vi "Write Ramp Current.vi"(8 "error in":errorcluster, 10 "Current_Ramp":dbl, 11 "69X_79X in":refnum<class "7976A.lvclass">) -> (0 "error out":errorcluster, 3 "69X_79X out":refnum<class "7976A.lvclass">)   [LabVIEW 2019, in "7976A.lvlib" / "7976A.lvclass"]
uses:
  Library/7976A.lvclass
  C:/Users/Public/Documents/Development/builds/Instruments/PowerSupply.lvlibp/Library/PowerSupply.lvclass
  builds/Instruments/PowerSupply.lvlibp/Library/PowerSupply.lvclass
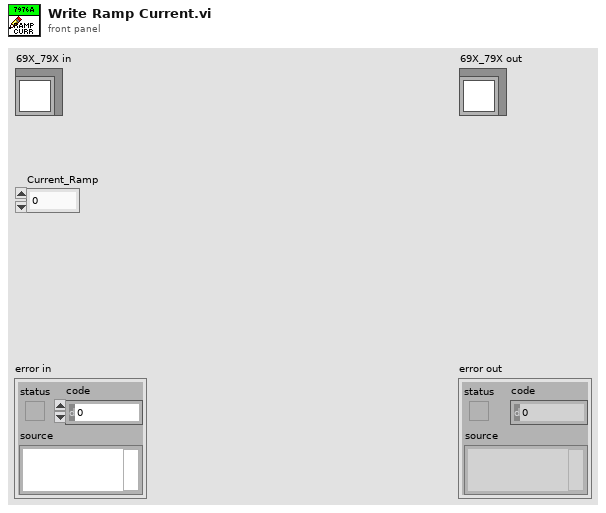
[diagram p1: front panel]
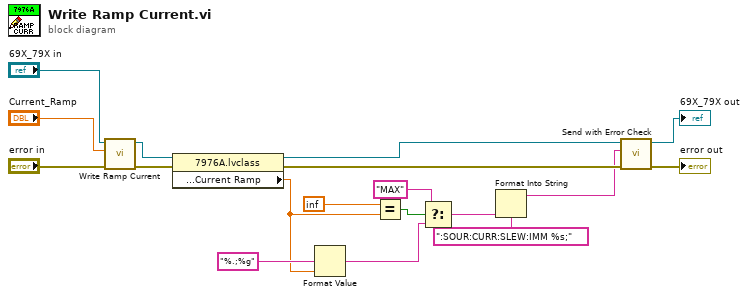
[diagram p0: block diagram]
diagram:
  n1 = call-parent "Write Ramp Current.vi"("error in"="error in", "Current_Ramp"="Current_Ramp", "PowerSupply in"="69X_79X in") -> ("error out"=w15:errorcluster, "PowerSupply out"=w11:refnum<class "7976A.lvclass">)  [unwired: 7 in]
  n2 = property class="7976A.lvclass"(reference=w11, error in=w15) -> (reference out=w10:refnum<class "7976A.lvclass">, error out=w12:errorcluster, "Accessors:Setting:Ramp:Current Ramp"=w6:dbl)
  n3 = Format Value(format string="%.;%g", value (0)=w6) -> (output string=w4:string)  [unwired: 1 in]
  n4 = Equal?(x=inf, y=w6) -> (x = y?=w5:bool)
  n5 = Select(t="MAX", s=w5, f=w4) -> (s? t:f=w3:string)
  n6 = Format Into String(format string=":SOUR:CURR:SLEW:IMM %s;", w3) -> (resulting string=w2:string)  [unwired: 2 in, 1 out]
  n7 = call "Send with Error Check.vi"("error in (no error)"=w12, "Command"=w2, "7976A in"=w10) -> ("error out"=→"error out":errorcluster, "7976A out"=→"69X_79X out":refnum<class "7976A.lvclass">)  [unwired: 7 in]
